vi "Read Key of Base DataType.vi"(5 "format string (%;%f)":string="%f", 7 "section":string, 8 "error in (no error)":errorcluster, 9 "type":variant, 10 "key (optional)":string, 11 "refnum":T1) -> (0 "error out":errorcluster, 1 "key-value":variant, 2 "found?":bool, 3 "refnum out":T1)   [LabVIEW 2017, in "INI++.lvlib"]
doc: "Reads a value associated with key in a specified section of the configuration data identified by refnum. If \"key\" input is not specified, the name of the variant object is used as the key. the \"found?\" output will be TRUE for compount objects (clusters) only if all elements (recursively) are found.\n\nFor example a Boolean named \"Enable\" with a value of TRUE would correspond to the key-value pair:\n\nEnable=TRUE\n\nNote: Special characters in section and key names will be escape-coded. These include the following: \\00-\\1F (non-printable chars); \"[\", \"]\", and \"=\" (INI syntax elements); \\FE (\"þ\") and \\FF (\"ÿ\") (legacy bracket encoding); Additionally, the escape character, \"\\\", will be escaped as \"\\\\\"."
uses:
  <vilib>/Utility/config.llb/Config Data RefNum.ctl
  <vilib>/Utility/Data Type/Type Definitions/Data Type.ctl
  <vilib>/Utility/config.llb/Read Key (String).vi
  <vilib>/Utility/config.llb/Read Key (Double).vi
  INI++.lvlib
  <vilib>/Utility/config.llb/Read Key (I32).vi
  <vilib>/Utility/config.llb/Read Key (U32).vi
  <vilib>/Utility/config.llb/Read Key (Path).vi
  <vilib>/Utility/config.llb/Read Key (Boolean).vi
  <vilib>/Utility/config.llb/NI_LVConfig.lvlib
  <vilib>/Utility/Data Type/NI_Data Type.lvlib
  _openG/_reuse_openG.lvlib
panel:
  in  "Ref for recursive call":refnum<vi>
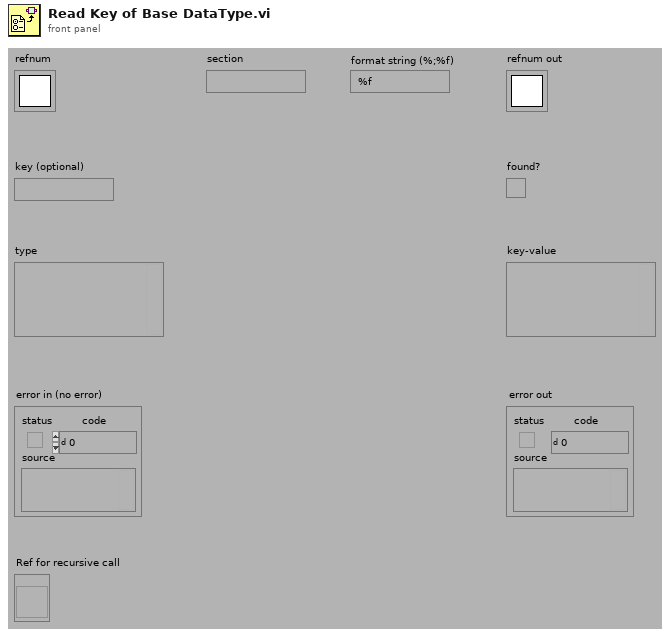
[diagram p1: front panel]
types:
  T1 = typedef "NI_LVConfig.lvlib/Config Data RefNum.ctl" = refnum<k1>
  T2 = typedef "NI_Data Type.lvlib/Data Type.ctl" = enum8{"Invalid Type", "Void", "I8", "I16", "I32", "I64", "U8", "U16", "U32", "U64", "Single Float", "Double Float", "Extended Float", "Single Complex", "Double Complex", "Extended Complex", "Enum U8", "Enum U16", "Enum U32", "Enum U64", "Single Float With Unit", "Double Float With Unit", "Extended Float With Unit", "Single Complex with Unit", "Double Complex with Unit", "Extended Complex with Unit", "Boolean", "String", "Path", "Picture", "Tag", "Array", "Cluster", "Variant", "LV Variant", "Waveform", "Timestamp", "Digital Waveform", "Digital Data", "ExpressData", "Refnum", "External Data", "VI", "Poly VI", "LabVIEW Class Instance", "Fixed Point"}
  T3 = typedef "Type Descriptor Enumeration__ogtk.ctl" = enum8{"<Null>", "I8", "I16", "I32", "I64", "U8", "U16", "U32", "U64", "SGL", "DBL", "EXT", "CSG", "CDB", "CXT", "0x0F", "0x10", "0x11", "0x12", "0x13", "0x14", "Enum U8", "Enum U16", "Enum U32", "Enum U64", "SGL PQ", "DBL PQ", "EXT PQ", "CSG PQ", "CDB PQ", "CXT PQ", "0x1F", "0x20", "Boolean", "0x22", "0x23", "0x24", "0x25", "0x26", "0x27", "0x28", "0x29", "0x2A", "0x2B", "0x2C", "0x2D", "0x2E", "0x2F", "String", "0x31", "Path", "Pict", "0x34", "0x35", "0x36", "DAQ", "0x38", "0x39", "0x3A", "0x3B", "0x3C", "0x3D", "0x3E", "0x3F", "Array", "0x41", "0x42", "0x43", "0x44", "0x45", "0x46", "0x47", "0x48", "0x49", "0x4A", "0x4B", "0x4C", "0x4D", "0x4E", "0x4F", "Cluster", "0x51", "0x52", "Variant", "Waveform", "0x55", "0x56", "0x57", "0x58", "0x59", "0x5A", "0x5B", "0x5C", "0x5D", "0x5E", "Fixed Point", "0x60", "0x61", "0x62", "0x63", "0x64", "0x65", "0x66", "0x67", "0x68", "0x69", "0x6A", "0x6B", "0x6C", "0x6D", "0x6E", "0x6F", "Refnum", "0x71", "0x72", "Set Collection", "Map Collection"}
  T4 = typedef "Type Descriptor__ogtk.ctl" = i16[]
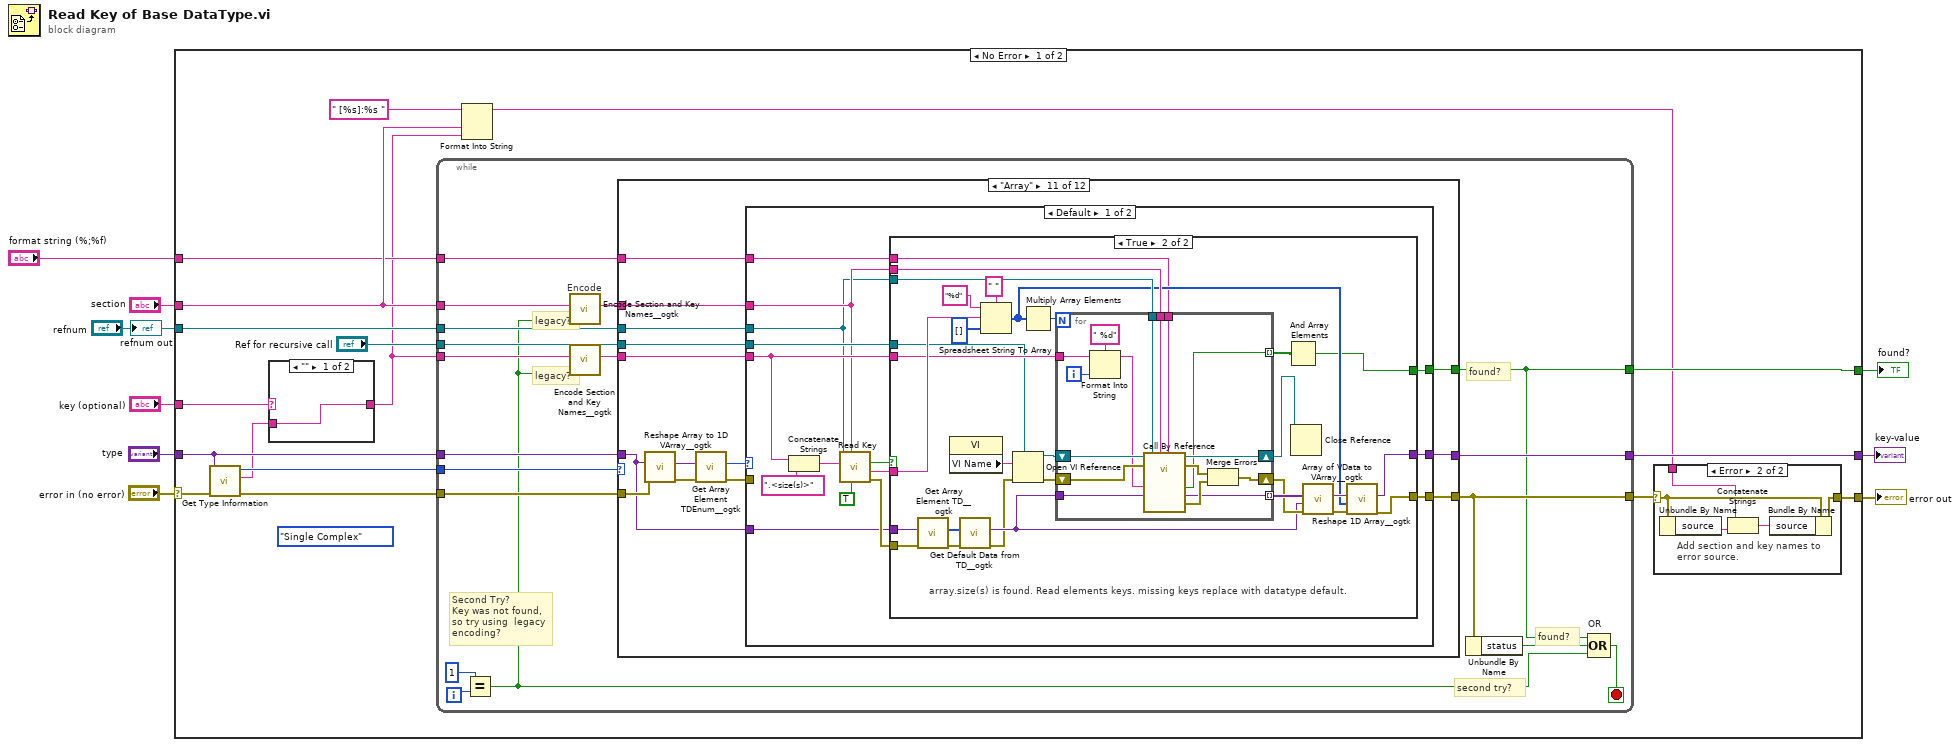
[diagram p0: block diagram]
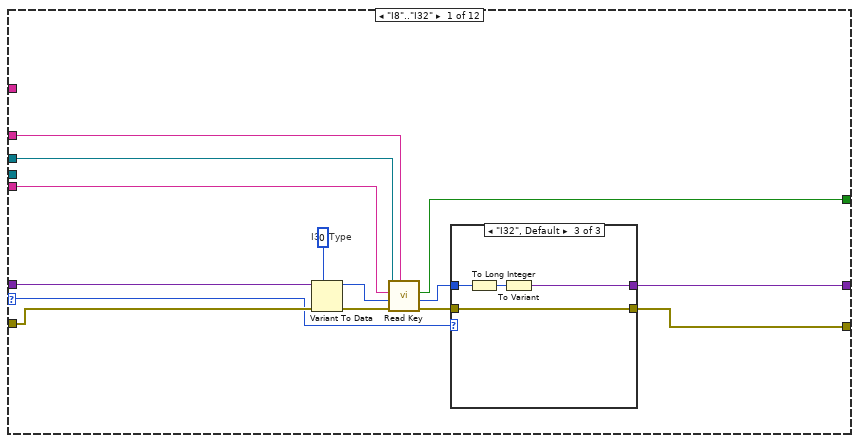
[diagram p3: hidden frame]
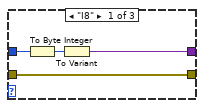
[diagram p4: hidden frame]
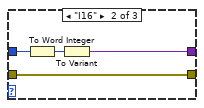
[diagram p5: hidden frame]
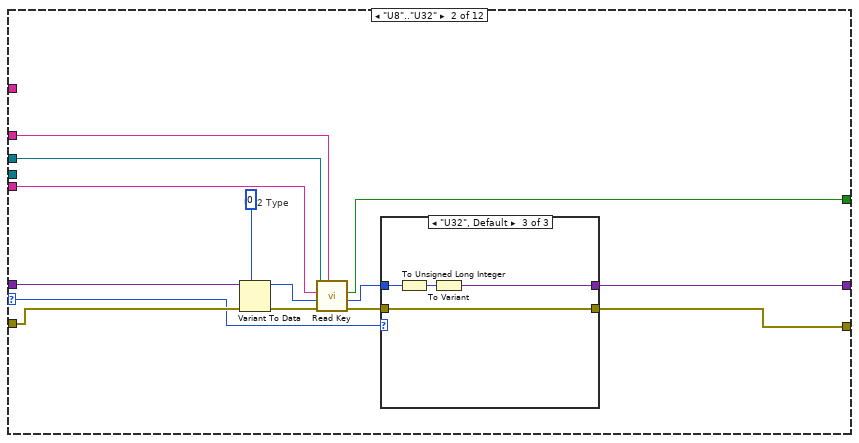
[diagram p6: hidden frame]
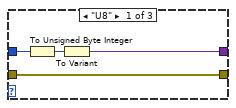
[diagram p7: hidden frame]
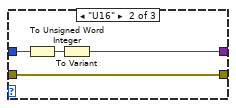
[diagram p8: hidden frame]
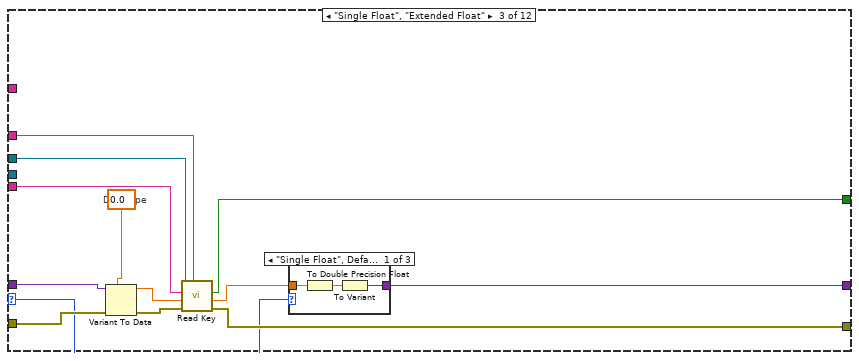
[diagram p9: hidden frame]
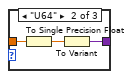
[diagram p10: hidden frame]
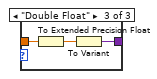
[diagram p11: hidden frame]
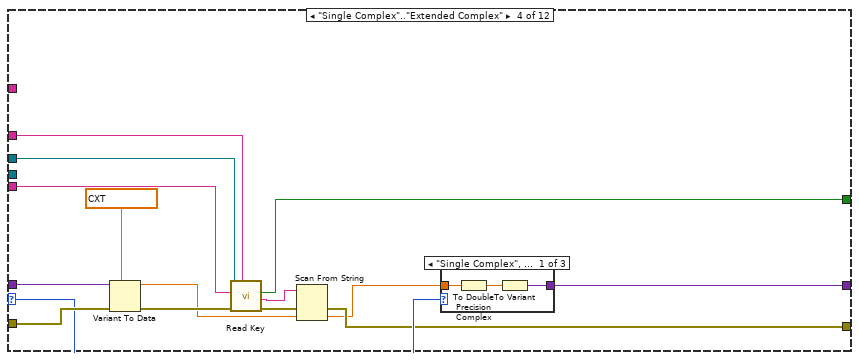
[diagram p12: hidden frame]
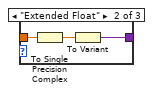
[diagram p13: hidden frame]
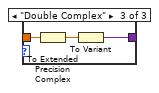
[diagram p14: hidden frame]
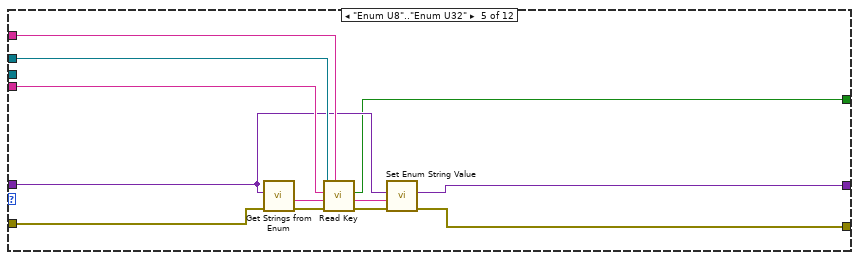
[diagram p15: hidden frame]
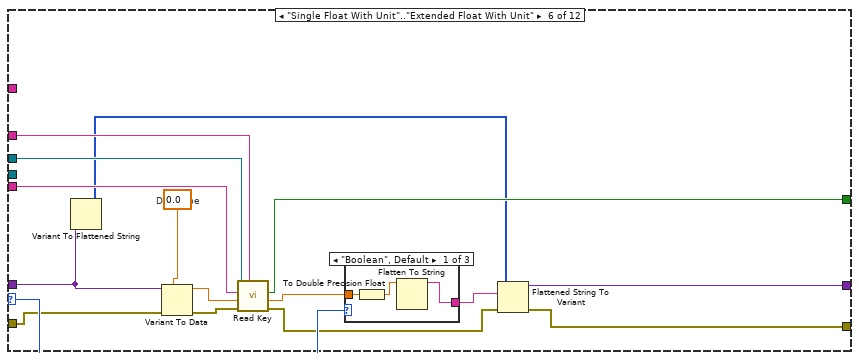
[diagram p16: hidden frame]
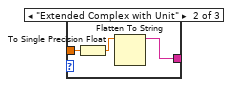
[diagram p17: hidden frame]
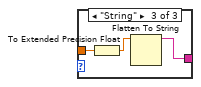
[diagram p18: hidden frame]
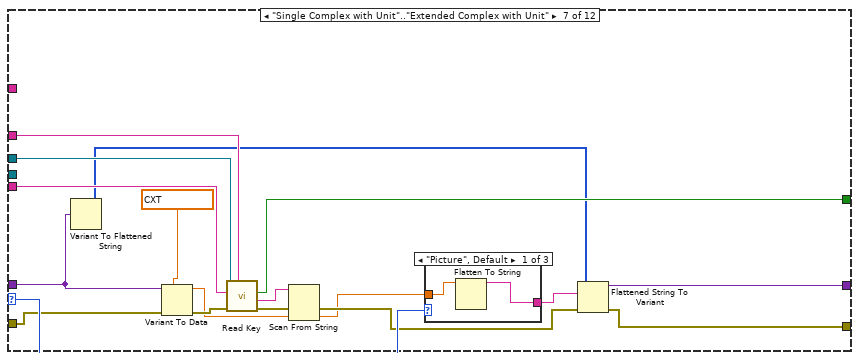
[diagram p19: hidden frame]
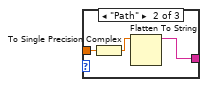
[diagram p20: hidden frame]
diagram:
  n1 = case shown="No Error" "error in (no error)" {
    selector: "error in (no error)" -> [w24 w410]
    tunnel: "refnum" -> [w26 _]
    tunnel: [w18 w410] -> w9
    tunnel: "type" -> [w22 _]
    tunnel: "key (optional)" -> [w12 _]
    tunnel: "section" -> [w15 _]
    tunnel: [w25 variant ("Variant")] -> w4
    tunnel: [w21 FALSE ("found?")] -> w2
    tunnel: "format string (%;%f)" -> [w14 _]
    frame No Error {
      (unwired) Data_Type."Single Complex" ("Type")
      n2 = call <vilib>:"Get Type Information.vi"("error in (no error)"=w24, "Variant"=w22) -> ("error out"=w23:errorcluster, "Name"=w10:string, "Type"=w13:T2)  [unwired: 5 in, 2 out]
      n3 = case shown="\"\"" w12 {
        selector: w12 -> [_ w28]
        tunnel: [w27 w28] -> w11
        tunnel: w10 -> [w27 _]
        frame "" {
        }
        frame Default {
        }
      }
      n4 = while {
        tunnel: w13 -> [w46]
        tunnel: w26 -> [w45]
        tunnel: [w44] -> w25
        tunnel: w23 -> [w43]
        tunnel: w22 -> [w42]
        tunnel: [w34] -> w21
        tunnel: "Ref for recursive call" -> [w41]
        tunnel: [w36] -> w19
        tunnel: w15 -> [w39]
        tunnel: w11 -> [w38]
        tunnel: w14 -> [w29]
        i -> [w33]
        stop <- w31 stop-if-true
        # "found?"
        # "found?"
        # "second try?"
        # "legacy?"
        # "legacy?"
        # "Second Try?\nKey was not found, so try using  legacy encoding?"
        # "Encode"
        n5 = Equal?(x=1, y=w33) -> (x = y?=w30:bool)
        n6 = call <userlib>:"Encode Section and Key Names__ogtk.vi"("use legacy encoding scheme? (FALSE)"=w30, "string"=w39) -> ("encoded string"=w40:string)  [unwired: 9 in]
        n7 = call <userlib>:"Encode Section and Key Names__ogtk.vi"("use legacy encoding scheme? (FALSE)"=w30, "string"=w38) -> ("encoded string"=w37:string)  [unwired: 9 in]
        n8 = case shown="\"Array\"" w46 {
          selector: w46 -> [w49 w75 w99 w126 _ w164 w193 _ _ _ _ _]
          tunnel: w42 -> [w59 w85 w110 w134 w147 w159 w189 w218 w230 w242 w246 w398]
          tunnel: w45 -> [w58 w84 w109 w133 w156 w171 w198 w217 w229 w241 w253 w401]
          tunnel: [w48 w73 w107 w124 w149 w161 w191 w215 w227 w239 w250 w392] -> w36
          tunnel: w43 -> [w56 w82 w106 w131 w153 w163 w192 w214 w226 w238 w256 w394]
          tunnel: w37 -> [w55 w81 w105 w130 w155 w169 w196 w213 w225 w237 w247 w400]
          tunnel: w40 -> [w54 w80 w104 w129 w154 w168 w195 w212 w224 w236 w248 w399]
          tunnel: [w47 w77 w101 w128 w146 w157 w187 w209 w223 w233 w251 w395] -> w44
          tunnel: [w52 w76 w100 w127 w145 w165 w194 w208 w220 w232 w249 w390] -> w34
          tunnel: w41 -> [_ _ _ _ _ _ _ _ _ _ w252 _]
          tunnel: w29 -> [_ _ _ _ _ _ _ _ _ _ w244 _]
          frame "I8".."I32" {
            # "I32 Type"
            n9 = Variant To Data(error in=w56, type=0, Variant=w59) -> (data=w53:i32, error out=w57:errorcluster)
            n10 = call-poly <vilib>:"Read Key.vi"("section"=w54, "error in (no error)"=w57, "default value"=w53, "key"=w55, "refnum"=w58) -> ("error out"=w51:errorcluster, "value"=w50:i32, "found?"=w52:bool)  [unwired: 3 in, 1 out]
            n11 = case shown="\"I32\", Default" w49 {
              tunnel: w50 -> [w64 w68 w72]
              tunnel: [w63 w67 w71] -> w47
              tunnel: w51 -> [w61 w65 w69]
              tunnel: [w61 w65 w69] -> w48
              frame "I8" {
                n12 = To Byte Integer(number=w64) -> (8bit integer=w62:i8)
                n13 = To Variant(anything=w62) -> (Variant=w63:variant)
              }
              frame "I16" {
                n14 = To Word Integer(number=w68) -> (16bit integer=w66:i16)
                n15 = To Variant(anything=w66) -> (Variant=w67:variant)
              }
              frame "I32", Default {
                n16 = To Long Integer(number=w72) -> (32bit integer=w70:i32)
                n17 = To Variant(anything=w70) -> (Variant=w71:variant)
              }
            }
          }
          frame "U8".."U32" {
            # "U32 Type"
            n18 = Variant To Data(error in=w82, type=u32 0, Variant=w85) -> (data=w79:u32, error out=w83:errorcluster)
            n19 = call-poly <vilib>:"Read Key.vi"("section"=w80, "error in (no error)"=w83, "default value"=w79, "key"=w81, "refnum"=w84) -> ("error out"=w74:errorcluster, "value"=w78:u32, "found?"=w76:bool)  [unwired: 3 in, 1 out]
            n20 = case shown="\"U32\", Default" w75 {
              tunnel: w78 -> [w90 w94 w98]
              tunnel: [w89 w93 w97] -> w77
              tunnel: w74 -> [w87 w91 w95]
              tunnel: [w87 w91 w95] -> w73
              frame "U8" {
                n21 = To Unsigned Byte Integer(number=w90) -> (unsigned 8bit integer=w88:u8)
                n22 = To Variant(anything=w88) -> (Variant=w89:variant)
              }
              frame "U16" {
                n23 = To Unsigned Word Integer(number=w94) -> (unsigned 16bit integer=w92:u16)
                n24 = To Variant(anything=w92) -> (Variant=w93:variant)
              }
              frame "U32", Default {
                n25 = To Unsigned Long Integer(number=w98) -> (unsigned 32bit integer=w96:u32)
                n26 = To Variant(anything=w96) -> (Variant=w97:variant)
              }
            }
          }
          frame "Single Float", "Extended Float" {
            # "DBL Type"
            n27 = Variant To Data(error in=w106, type=0.0, Variant=w110) -> (data=w103:dbl, error out=w108:errorcluster)
            n28 = call-poly <vilib>:"Read Key.vi"("section"=w104, "error in (no error)"=w108, "default value"=w103, "key"=w105, "refnum"=w109) -> ("error out"=w107:errorcluster, "value"=w102:dbl, "found?"=w100:bool)  [unwired: 3 in, 1 out]
            n29 = case shown="\"Single Float\", Default" w99 {
              tunnel: w102 -> [w114 w117 w120]
              tunnel: [w113 w116 w119] -> w101
              frame "Single Float", Default {
                n30 = To Double Precision Float(number=w114) -> (double precision float=w112:dbl)
                n31 = To Variant(anything=w112) -> (Variant=w113:variant)
              }
              frame "U64" {
                n32 = To Single Precision Float(number=w117) -> (single precision float=w115:sgl)
                n33 = To Variant(anything=w115) -> (Variant=w116:variant)
              }
              frame "Double Float" {
                n34 = To Extended Precision Float(1:w120) -> (0:w118:ext)
                n35 = To Variant(anything=w118) -> (Variant=w119:variant)
              }
            }
          }
          frame "Single Complex".."Extended Complex" {
            # "CXT Type"
            n36 = Variant To Data(error in=w131, type=cxt 0.0+0.0i, Variant=w134) -> (data=w122:cxt, error out=w132:errorcluster)
            n37 = call-poly <vilib>:"Read Key.vi"("section"=w129, "error in (no error)"=w132, "key"=w130, "refnum"=w133) -> ("error out"=w125:errorcluster, "value"=w123:string, "found?"=w127:bool)  [unwired: 4 in, 1 out]
            n38 = Scan From String(input string=w123, error in=w125, default 1=w122) -> (error out=w124:errorcluster, output 1=w121:cxt)  [unwired: 2 in, 2 out]
            n39 = case shown="\"Single Complex\", Default" w126 {
              tunnel: w121 -> [w138 w141 w144]
              tunnel: [w137 w140 w143] -> w128
              frame "Single Complex", Default {
                n40 = To Double Precision Complex(1:w138) -> (0:w136:cdb)
                n41 = To Variant(anything=w136) -> (Variant=w137:variant)
              }
              frame "Extended Float" {
                n42 = To Single Precision Complex(1:w141) -> (0:w139:csg)
                n43 = To Variant(anything=w139) -> (Variant=w140:variant)
              }
              frame "Double Complex" {
                n44 = To Extended Precision Complex(1:w144) -> (0:w142:cxt)
                n45 = To Variant(anything=w142) -> (Variant=w143:variant)
              }
            }
          }
          frame "Enum U8".."Enum U32" {
            n46 = call "Get Strings from Enum.vi"("error in (no error)"=w153, "Enum"=w147) -> ("error out"=w152:errorcluster, "String Value"=w151:string)  [unwired: 6 in, 2 out]
            n47 = call-poly <vilib>:"Read Key.vi"("section"=w154, "error in (no error)"=w152, "default value"=w151, "key"=w155, "refnum"=w156) -> ("error out"=w150:errorcluster, "value"=w148:string, "found?"=w145:bool)  [unwired: 3 in, 1 out]
            n48 = call "Set Enum String Value.vi"("error in (no error)"=w150, "String Value"=w148, "Default Enum Value"=w147) -> ("error out"=w149:errorcluster, "Enum"=w146:variant)  [unwired: 7 in]
          }
          frame "Single Float With Unit".."Extended Float With Unit" {
            # "DBL Type"
            n49 = Variant To Flattened String(Variant=w159) -> (1:w158:i16[])  [unwired: 1 out]
            n50 = Variant To Data(error in=w163, type=0.0, Variant=w159) -> (data=w167:dbl, error out=w170:errorcluster)
            n51 = call-poly <vilib>:"Read Key.vi"("section"=w168, "error in (no error)"=w170, "default value"=w167, "key"=w169, "refnum"=w171) -> ("error out"=w162:errorcluster, "value"=w166:dbl, "found?"=w165:bool)  [unwired: 3 in, 1 out]
            n52 = case shown="\"Boolean\", Default" w164 {
              tunnel: w166 -> [w175 w178 w181]
              tunnel: [w174 w176 w179] -> w160
              frame "Boolean", Default {
                n53 = To Double Precision Float(number=w175) -> (double precision float=w173:dbl)
                n54 = Flatten To String(anything=w173) -> (data string=w174:string)  [unwired: 3 in, 2 out]
              }
              frame "Extended Complex with Unit" {
                n55 = To Single Precision Float(number=w178) -> (single precision float=w177:sgl)
                n56 = Flatten To String(anything=w177) -> (data string=w176:string)  [unwired: 3 in, 2 out]
              }
              frame "String" {
                n57 = To Extended Precision Float(1:w181) -> (0:w180:ext)
                n58 = Flatten To String(anything=w180) -> (data string=w179:string)  [unwired: 3 in, 2 out]
              }
            }
            n59 = Flattened String To Variant(4:w162, 6:w160, 7:w158) -> (0:w161:errorcluster, 3:w157:variant)
          }
          frame "Single Complex with Unit".."Extended Complex with Unit" {
            # "CXT Type"
            n60 = Variant To Flattened String(Variant=w189) -> (1:w188:i16[])  [unwired: 1 out]
            n61 = Variant To Data(error in=w192, type=cxt 0.0+0.0i, Variant=w189) -> (data=w183:cxt, error out=w197:errorcluster)
            n62 = call-poly <vilib>:"Read Key.vi"("section"=w195, "error in (no error)"=w197, "key"=w196, "refnum"=w198) -> ("error out"=w185:errorcluster, "value"=w184:string, "found?"=w194:bool)  [unwired: 4 in, 1 out]
            n63 = Scan From String(input string=w184, error in=w185, default 1=w183) -> (error out=w186:errorcluster, output 1=w182:cxt)  [unwired: 2 in, 2 out]
            n64 = case shown="\"Picture\", Default" w193 {
              tunnel: w182 -> [w201 w204 w207]
              tunnel: [w200 w202 w205] -> w190
              frame "Picture", Default {
                n65 = Flatten To String(anything=w201) -> (data string=w200:string)  [unwired: 3 in, 2 out]
              }
              frame "Path" {
                n66 = To Single Precision Complex(1:w204) -> (0:w203:csg)
                n67 = Flatten To String(anything=w203) -> (data string=w202:string)  [unwired: 3 in, 2 out]
              }
              frame "Tag" {
                n68 = To Extended Precision Complex(1:w207) -> (0:w206:cxt)
                n69 = Flatten To String(anything=w206) -> (data string=w205:string)  [unwired: 3 in, 2 out]
              }
            }
            n70 = Flattened String To Variant(4:w186, 6:w190, 7:w188) -> (0:w191:errorcluster, 3:w187:variant)
          }
          frame "Boolean" {
            # "Boolean Type"
            n71 = Variant To Data(error in=w214, type=FALSE, Variant=w218) -> (data=w211:bool, error out=w216:errorcluster)
            n72 = call-poly <vilib>:"Read Key.vi"("section"=w212, "error in (no error)"=w216, "default value"=w211, "key"=w213, "refnum"=w217) -> ("error out"=w215:errorcluster, "value"=w210:bool, "found?"=w208:bool)  [unwired: 3 in, 1 out]
            n73 = To Variant(anything=w210) -> (Variant=w209:variant)
          }
          frame "String", "Tag" {
            # "String Type"
            n74 = Variant To Data(error in=w226, type="", Variant=w230) -> (data=w221:string, error out=w228:errorcluster)
            n75 = call-poly <vilib>:"Read Key.vi"("section"=w224, "error in (no error)"=w228, "default value"=w221, "key"=w225, "refnum"=w229) -> ("error out"=w227:errorcluster, "value"=w222:string, "found?"=w220:bool)  [unwired: 3 in, 1 out]
            n76 = To Variant(anything=w222) -> (Variant=w223:variant)
          }
          frame "Path" {
            # "Path Type"
            n77 = Variant To Data(error in=w238, type=path "", Variant=w242) -> (data=w235:path, error out=w240:errorcluster)
            n78 = call-poly <vilib>:"Read Key.vi"("section"=w236, "error in (no error)"=w240, "default value"=w235, "key"=w237, "refnum"=w241) -> ("error out"=w239:errorcluster, "value"=w234:path, "found?"=w232:bool)  [unwired: 3 in, 1 out]
            n79 = To Variant(anything=w234) -> (Variant=w233:variant)
          }
          frame "Array" {
            n80 = call <userlib>:"Reshape Array to 1D VArray__ogtk.vi"("error in (no error)"=w256, "MultiD Array"=w246) -> ("error out"=w257:errorcluster, "1D VArray"=w245:variant)  [unwired: 7 in, 1 out]
            n81 = call <userlib>:"Get Array Element TDEnum__ogtk.vi"("error in (no error)"=w257, "Array"=w245) -> ("error out"=w254:errorcluster, "Element Type"=w255:T3)  [unwired: 8 in]
            n82 = case shown="Default" w255 {
              selector: w255 -> [_ w336]
              tunnel: w254 -> [_ w346]
              tunnel: w246 -> [w267 w324]
              tunnel: w248 -> [w265 w347]
              tunnel: w253 -> [w264 w348]
              tunnel: w247 -> [w268 w349]
              tunnel: w252 -> [w266 _]
              tunnel: [w262 w323] -> w251
              tunnel: [w261 errorcluster {"status"=FALSE, "code"=0, "source"=""} ("error out")] -> w250
              tunnel: [w260 w345] -> w249
              tunnel: w244 -> [w258 w321]
              frame Default {
                n83 = Concatenate Strings(w268, ".<size(s)>" ("Substring")) -> (w271:string)
                n84 = call-poly <vilib>:"Read Key.vi"("read raw string? (F)"=TRUE, "section"=w265, "key"=w271, "refnum"=w264) -> ("error out"=w269:errorcluster, "value"=w270:string, "found?"=w259:bool)  [unwired: 4 in, 1 out]
                n85 = case shown="True" w259 {
                  tunnel: w270 -> [_ w302]
                  tunnel: w269 -> [_ w278]
                  tunnel: w268 -> [_ w297]
                  tunnel: w267 -> [w274 w296]
                  tunnel: w266 -> [_ w295]
                  tunnel: w265 -> [_ w293]
                  tunnel: w264 -> [_ w292]
                  tunnel: [w274 w285] -> w262
                  tunnel: [errorcluster {"status"=FALSE, "code"=0, "source"=""} ("error out") w284] -> w261
                  tunnel: [FALSE w282] -> w260
                  tunnel: w258 -> [_ w276]
                  frame False {
                    # "array size(s) not found. Ignore element keys (if any) and return input array"
                  }
                  frame True {
                    # "array.size(s) is found. Read elements keys. missing keys replace with datatype default."
                    n86 = call <userlib>:"Get Array Element TD__ogtk.vi"("error in (no error)"=w278, "Array"=w296) -> ("error out"=w280:errorcluster, "Type Descriptor"=w281:T4)  [unwired: 8 in]
                    n87 = property class="VI"() -> ("VI Name"=w299:string)  [unwired: 2 in, 2 out]
                    n88 = call <userlib>:"Get Default Data from TD__ogtk.vi"("error in (no error)"=w280, "Type Descriptor"=w281) -> ("error out"=w277:errorcluster, "Default VData"=w279:variant)  [unwired: 8 in]
                    n89 = Spreadsheet String To Array(delimiter (Tab)=" ", format string="%d", spreadsheet string=w302, array type (2D Dbl)=u32[] [] ("Array Constant")) -> (array=w286:u32[])
                    n90 = Open VI Reference(type specifier VI Refnum (for type only)=w295, vi path=w299, error in (no error)=w277) -> (vi reference=w294:refnum<vi>, error out=w298:errorcluster)  [unwired: 3 in]
                    n91 = Multiply Array Elements(1:w286) -> (0:w300:u32)
                    n92 = for {
                      N: w300 -> [_]
                      shift-right: [w314] -> w289
                      shift-left: w298 -> [w311]
                      shift-right: [w315] -> w291
                      shift-left: w294 -> [w313]
                      tunnel: w297 -> [w318]
                      tunnel: w279 -> [w312]
                      tunnel: w293 -> [w309]
                      tunnel: w292 -> [w308]
                      tunnel: [w307] -> w290 mode=indexing
                      tunnel: [w306] -> w283 mode=indexing
                      tunnel: w276 -> [w305]
                      i -> [w319]
                      n93 = Format Into String(format string=" %d" ("Format String"), initial string=w318, w319) -> (resulting string=w310:string)  [unwired: 1 in, 1 out]
                      n94 = call-by-ref "?"(reference=w313, error in=w311, "format string (%;%f"=w305, "section"=w309, "type"=w312, "key (optional)"=w310, "refnum"=w308) -> (reference out=w315:refnum<vi>, error out=w317:errorcluster, "error out"=w316:errorcluster, "key-value"=w307:variant, "found?"=w306:bool)  [unwired: 3 in, 1 out]
                      n95 = Merge Errors(w317, w316) -> (w314:errorcluster)
                    }
                    n96 = And Array Elements(Boolean array=w283) -> (logical AND=w282:bool)
                    n97 = Close Reference(reference=w291) -> ()  [unwired: 1 in, 1 out]
                    n98 = call <userlib>:"Array of VData to VArray__ogtk.vi"("error in (no error)"=w289, "Element Type (when empty)"=w279, "1D Array of VData"=w290) -> ("error out"=w288:errorcluster, "VArray"=w287:variant)  [unwired: 7 in]
                    n99 = call <userlib>:"Reshape 1D Array__ogtk.vi"("error in (no error)"=w288, "Size(s)"=w286, "1D Array"=w287) -> ("error out"=w284:errorcluster, "Reshaped VArray"=w285:variant)  [unwired: 7 in]
                  }
                }
              }
              frame "I8".."I32", "U8".."U32", "SGL".."EXT", "SGL PQ".."EXT PQ" {
                n100 = call-poly <vilib>:"Read Key.vi"("section"=w347, "error in (no error)"=w346, "key"=w349, "refnum"=w348) -> ("error out"=w344:errorcluster, "value"=w350:string, "found?"=w345:bool)  [unwired: 4 in, 1 out]
                n101 = Scan From String(format string="<size(s)=%[\\s0-9]> " ("regular expression"), input string=w350, error in=w344) -> (remaining string=w337:string, error out=w327:errorcluster, output 1=w342:string)  [unwired: 2 in, 1 out]
                n102 = Variant To Flattened String(Variant=w324) -> (data string=w329:string, 1:w330:i16[])
                n103 = Spreadsheet String To Array(delimiter (Tab)=" ", format string="%d", spreadsheet string=w342, array type (2D Dbl)=u32[] []) -> (array=w343:u32[])
                n104 = Type Cast(x=w343) -> (*(type *) &x=w334:string)  [unwired: 1 in]
                n105 = Spreadsheet String To Array(delimiter (Tab)=" ", format string=w321, spreadsheet string=w337, array type (2D Dbl)=dbl[] []) -> (array=w335:dbl[])
                n106 = case shown="\"SGL\", \"SGL PQ\"" w336 {
                  tunnel: w335 -> [_ w357 w361 w365 w369 w373 w377 w381 w383 w387]
                  tunnel: [w352 w355 w359 w363 w367 w371 w375 w379 w385 w389] -> w332
                  tunnel: ["" w354 w358 w362 w366 w370 w374 w378 w384 w388] -> w331
                  tunnel: w334 -> [_ w354 w358 w362 w366 w370 w374 w378 w384 w388]
                  tunnel: w329 -> [w352 _ _ _ _ _ _ _ _ _]
                  frame Default {
                  }
                  frame "I8" {
                    n107 = To Byte Integer(number=w357) -> (8bit integer=w356:i8[])
                    n108 = Type Cast(x=w356) -> (*(type *) &x=w355:string)  [unwired: 1 in]
                  }
                  frame "I16" {
                    n109 = To Word Integer(number=w361) -> (16bit integer=w360:i16[])
                    n110 = Type Cast(x=w360) -> (*(type *) &x=w359:string)  [unwired: 1 in]
                  }
                  frame "I32" {
                    n111 = To Long Integer(number=w365) -> (32bit integer=w364:i32[])
                    n112 = Type Cast(x=w364) -> (*(type *) &x=w363:string)  [unwired: 1 in]
                  }
                  frame "U8" {
                    n113 = To Unsigned Byte Integer(number=w369) -> (unsigned 8bit integer=w368:u8[])
                    n114 = Type Cast(x=w368) -> (*(type *) &x=w367:string)  [unwired: 1 in]
                  }
                  frame "U16" {
                    n115 = To Unsigned Word Integer(number=w373) -> (unsigned 16bit integer=w372:u16[])
                    n116 = Type Cast(x=w372) -> (*(type *) &x=w371:string)  [unwired: 1 in]
                  }
                  frame "U32" {
                    n117 = To Unsigned Long Integer(number=w377) -> (unsigned 32bit integer=w376:u32[])
                    n118 = Type Cast(x=w376) -> (*(type *) &x=w375:string)  [unwired: 1 in]
                  }
                  frame "SGL", "SGL PQ" {
                    n119 = To Single Precision Float(number=w381) -> (single precision float=w380:sgl[])
                    n120 = Type Cast(x=w380) -> (*(type *) &x=w379:string)  [unwired: 1 in]
                  }
                  frame "DBL", "DBL PQ" {
                    n121 = To Double Precision Float(number=w383) -> (double precision float=w382:dbl[])
                    n122 = Type Cast(x=w382) -> (*(type *) &x=w385:string)  [unwired: 1 in]
                  }
                  frame "EXT", "EXT PQ" {
                    n123 = To Extended Precision Float(1:w387) -> (0:w386:ext[])
                    n124 = Type Cast(x=w386) -> (*(type *) &x=w389:string)  [unwired: 1 in]
                  }
                }
                n125 = Concatenate Strings(w331, w332) -> (w333:string)
                n126 = Flattened String To Variant(4:w327, 6:w333, 7:w330) -> (0:w326:errorcluster, 3:w325:variant)
                n127 = Select(t=w324, s=w326, f=w325) -> (s? t:f=w323:variant)
              }
            }
          }
          frame Default {
            n128 = Variant To Flattened String(Variant=w398) -> (data string=w397:string, 1:w391:i16[])
            n129 = call-poly <vilib>:"Read Key.vi"("section"=w399, "error in (no error)"=w394, "default value"=w397, "key"=w400, "refnum"=w401) -> ("error out"=w393:errorcluster, "value"=w396:string, "found?"=w390:bool)  [unwired: 3 in, 1 out]
            n130 = Flattened String To Variant(4:w393, 6:w396, 7:w391) -> (0:w392:errorcluster, 3:w395:variant)
          }
        }
        n131 = Unbundle By Name(w36) -> ("status"=w35:bool)
        n132 = Compound Arithmetic op=OR "OR"(w34, w35, w30) -> (w31:bool)
      }
      n133 = Format Into String(format string=" [%s]:%s " ("Format String"), w15, w11) -> (resulting string=w16:string)  [unwired: 2 in, 1 out]
      n134 = case shown="Error" w19 {
        selector: w19 -> [w402 w407]
        tunnel: [w402 w406] -> w18
        tunnel: w16 -> [_ w403]
        frame No Error {
        }
        frame Error {
          # "Add section and key names to\nerror source."
          n135 = Unbundle By Name(w407) -> ("source"=w404:string)
          n136 = Concatenate Strings(w403, w404) -> (w405:string)
          n137 = Bundle By Name(cluster=w407, "source"=w405) -> (w406:errorcluster)
        }
      }
    }
    frame Error {
    }
  }
  "error out" <- w9
  "key-value" <- w4
  "found?" <- w2
  "refnum out" <- "refnum"
